vi "Shutdown Thread.vi"(8 "error in (no error)":errorcluster, 11 "Thread in":refnum<class "Thread.lvclass">) -> (0 "error out":errorcluster, 3 "Thread out":refnum<class "Thread.lvclass">)   [LabVIEW 2019, in "DSF Core.lvlib" / "Thread.lvclass"]
uses:
  Thread.lvclass
  Thread.lvclass/Thread.ctl
  <vilib>/NI/Memory Manager/Classes/Pointer/Pointer.lvclass/Pointer.ctl
  Thread Command.ctl
  <vilib>/NI/Memory Manager/Classes/Pointer/Read.vi
  <vilib>/NI/Memory Manager/Classes/Pointer/Read U8.vi
  <vilib>/NI/Memory Manager/Classes/Pointer/Write.vi
  <vilib>/NI/Memory Manager/Classes/Pointer/Write Bool.vi
  <vilib>/NI/Memory Manager/Classes/Pointer/Read (No Check).vi
  <vilib>/NI/Memory Manager/Classes/Pointer/Read (No Check) U8.vi
  <vilib>/NI/Memory Manager/Classes/Pointer/Check Move.vi
  <vilib>/NI/Memory Manager/Classes/Pointer/Write (No Check).vi
  <vilib>/NI/Memory Manager/Classes/Pointer/Write (No Check) Bool.vi
  <vilib>/NI/Memory Manager/Classes/Pointer/Get Address.vi
  <vilib>/NI/Memory Manager/Classes/Pointer/Check Null Pointer.vi
  <vilib>/NI/Memory Manager/Classes/Pointer/Check Count.vi
  <vilib>/NI/Memory Manager/Classes/Pointer/Check Bounds (Power of 2).vi
  <vilib>/NI/Memory Manager/Classes/Pointer/Errors.vi
  <vilib>/NI/Memory Manager/Classes/Pointer/Null Pointer.vi
  <vilib>/NI/Memory Manager/Classes/Pointer/Is Null.vi
  <vilib>/NI/Memory Manager/Classes/Pointer/Get Size.vi
  <vilib>/NI/Memory Manager/Classes/Pointer/Out of Bounds.vi
  <vilib>/NI/Memory Manager/Classes/Pointer/Check Bounds.vi
  <vilib>/NI/Memory Manager/Classes/Pointer/Create Error.vi
  <vilib>/NI/Memory Manager/VIs/Write String to Source.vi
  <vilib>/NI/Memory Manager/Classes/Pointer/Write Pointer Size to Error.vi
  <vilib>/NI/Memory Manager/VIs/Write Numeric to Source.vi
  <vilib>/NI/Memory Manager/VIs/Write Numeric Scalar to Source (Base10 U64).vi
  <vilib>/NI/Memory Manager/Classes/Pointer/Check Bounds (Pointer).vi
  <vilib>/NI/Memory Manager/Classes/Pointer/Check Bounds (Buffer).vi
  <vilib>/NI/Memory Manager/VIs/New Error Cluster.vi
  <vilib>/NI/Memory Manager/VIs/New Error Cluster (512B).vi
  <vilib>/NI/Memory Manager/VIs/Set Error Status.vi
  <vilib>/NI/Memory Manager/VIs/Set Error Code.vi
  <vilib>/NI/Memory Manager/VIs/Set Error Source.vi
  <vilib>/NI/Memory Manager/Constants/Constants.vi
  <vilib>/NI/Memory Manager/Constants/Library Name.vi
  <vilib>/NI/Memory Manager/Classes/Pointer/Pointer Error Info.vi
  <vilib>/NI/Memory Manager/Constants/Pointer Class Name.vi
  <vilib>/NI/Memory Manager/Classes/Pointer/Buffer Underflow.vi
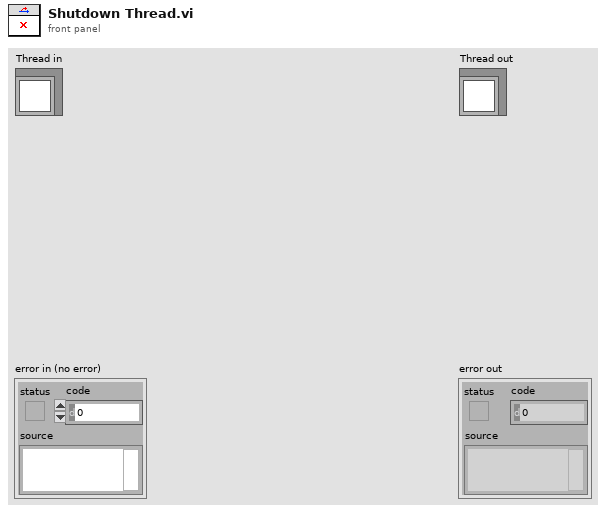
[diagram p1: front panel]
types:
  T1 = typedef "DSF Core.lvlib/Thread.lvclass/Thread State.ctl" = enum8{"Idle", "Running", "Error", "Shut Down"}
  T2 = typedef "DSF Core.lvlib/Thread.lvclass/Thread Command.ctl" = enum8{"Run", "Shutdown"}
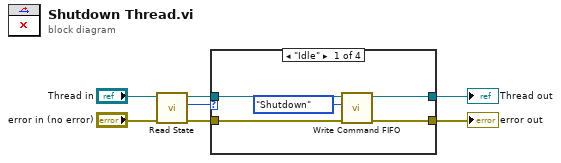
[diagram p0: block diagram]
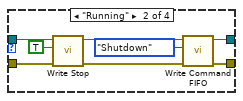
[diagram p2: hidden frame]
diagram:
  n1 = call "Read State.vi"("error in (no error)"="error in (no error)", "Thread in"="Thread in") -> ("error out"=w6:errorcluster, "state"=w1:T1, "Thread out"=w7:refnum<class "Thread.lvclass">)  [unwired: 7 in]
  n2 = case shown="\"Idle\"" w1 {
    tunnel: w7 -> [w12 w20 w22 w23]
    tunnel: w6 -> [w11 w19 w21 w24]
    tunnel: [w10 w14 w22 w23] -> w3
    tunnel: [w9 w15 w21 w24] -> w2
    frame "Idle" {
      n3 = call "Write Command FIFO.vi"("error in (no error)"=w11, "command"=Thread_Command."Shutdown", "Thread in"=w12) -> ("error out"=w9:errorcluster, "Thread out"=w10:refnum<class "Thread.lvclass">)  [unwired: 5 in, 2 out]
    }
    frame "Running" {
      n4 = call "Write Stop.vi"("error in (no error)"=w19, "stop"=TRUE, "Thread in"=w20) -> ("error out"=w16:errorcluster, "Thread out"=w13:refnum<class "Thread.lvclass">)  [unwired: 7 in]
      n5 = call "Write Command FIFO.vi"("error in (no error)"=w16, "command"=Thread_Command."Shutdown", "Thread in"=w13) -> ("error out"=w15:errorcluster, "Thread out"=w14:refnum<class "Thread.lvclass">)  [unwired: 5 in, 2 out]
    }
    frame "Error" {
    }
    frame "Shut Down" {
    }
  }
  "error out" <- w2
  "Thread out" <- w3
